vi "FPGA Target Approach Retraction1.vi"() -> ()   [LabVIEW 2013]
uses:
  <vilib>/eio/EIONode/EIONode.xnode
  <vilib>/rvi/eio/common/nirviEmuTemplateMethod_errors.vi
panel:
  out "FPGA Output Voltage":fxp<+/-,64,32>
  out "Z Fine Indicator":fxp<+/-,40,30>
  out "Counter Indicator":i32
  in  "Z Fine Output":fxp<+/-,40,30>
  in  "Counter Output":i32
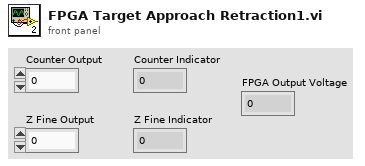
[diagram p1: front panel]
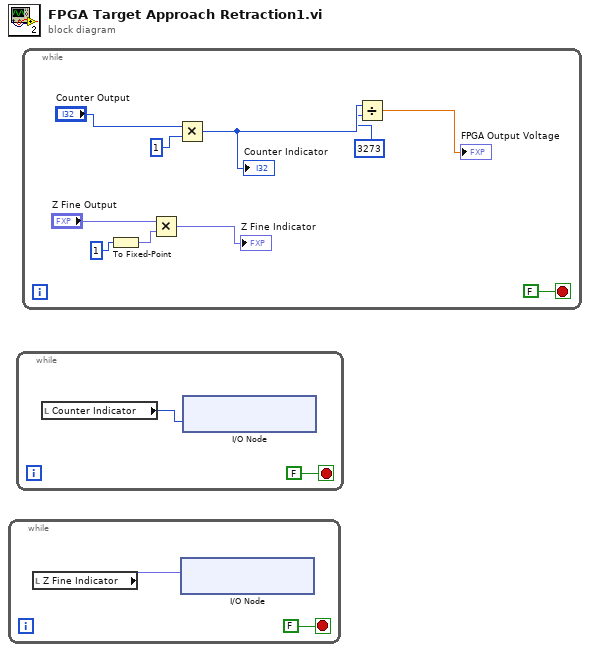
[diagram p0: block diagram]
diagram:
  n1 = while {
    stop <- FALSE stop-if-true
    n2 = local read "Z Fine Indicator"() -> (w1:fxp<+/-,40,30>)
    n3 = xnode "I/O Node"("Connector0/AO2"=w1) -> ()  [unwired: 1 in, 1 out]
  }
  n4 = while {
    stop <- FALSE stop-if-true
    n5 = local read "Counter Indicator"() -> (w3:i32)
    n6 = xnode "I/O Node"("Connector0/AO7"=w3) -> ()  [unwired: 1 in, 1 out]
  }
  n7 = while {
    stop <- FALSE stop-if-true
    n8 = To Fixed-Point(number=1) -> (fixed-point=w9:fxp<+/-,32,32>)  [unwired: 1 in]
    n9 = Multiply(x="Z Fine Output", y=w9) -> (x*y=→"Z Fine Indicator":fxp<+/-,64,62>)
    n10 = Multiply(x="Counter Output", y=1) -> (x*y=w8:i32)
    "Counter Indicator" <- w8
    n11 = Divide(x=w8, y=3273) -> (x/y=→"FPGA Output Voltage":dbl)
  }
